vi "Read Trigger Status.vi"(8 "error in (no error)":errorcluster, 11 "MSOX6004 in":refnum<class "MSOX6004.lvclass">) -> (0 "error out":errorcluster, 2 "Triggered?":bool, 3 "MSOX6004 out":refnum<class "MSOX6004.lvclass">)   [LabVIEW 2018, in "MSOX6004.lvlib" / "MSOX6004.lvclass"]
doc: "This Override inquired the Trigger status of the Oscope. It is meant to provide trigger status (any trigger)."
uses:
  MSOX6004.lvclass
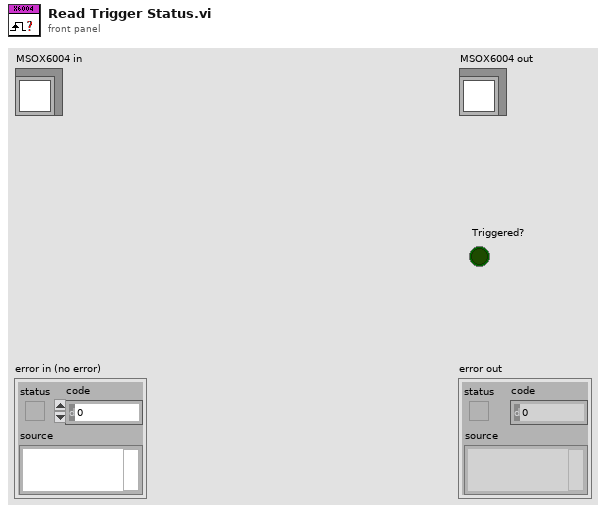
[diagram p1: front panel]
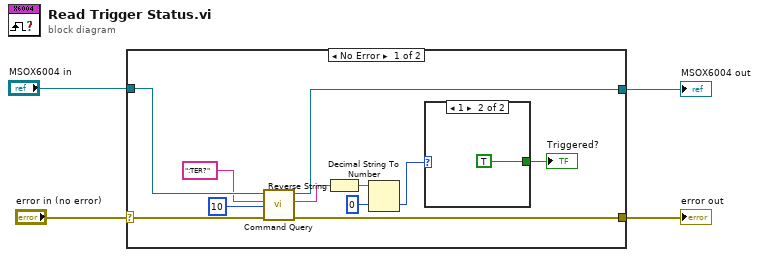
[diagram p0: block diagram]
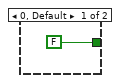
[diagram p2: hidden frame]
diagram:
  n1 = case shown="No Error" "error in (no error)" {
    selector: "error in (no error)" -> [w15 w18]
    tunnel: "MSOX6004 in" -> [w14 w19]
    tunnel: [w11 w19] -> w2
    tunnel: [w10 w18] -> w1
    frame No Error {
      n2 = call "Command Query.vi"("error in (no error)"=w15, "Delay (ms)"=u32 10, "Command"=":TER?", "MSOX6004 in"=w14) -> ("error out"=w10:errorcluster, "Response"=w5:string, "MSOX6004 out"=w11:refnum<class "MSOX6004.lvclass">)  [unwired: 5 in]
      n3 = Reverse String(1:w5) -> (0:w6:string)
      n4 = Decimal String To Number(string=w6, default (0L)=u16 0) -> (number=w8:u16)  [unwired: 1 in, 1 out]
      n5 = case shown="1" w8 {
        tunnel: [FALSE TRUE] -> w7
        frame 0, Default {
        }
        frame 1 {
        }
      }
      "Triggered?" <- w7
    }
    frame Error {
    }
  }
  "error out" <- w1
  "MSOX6004 out" <- w2
